vi "json_ltrim.vi"(10 "offset (0)":i32, 11 "data":string) -> (3 "left trim whitespace":string)   [LabVIEW 2017]
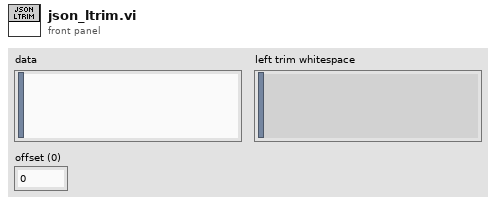
[diagram p1: front panel]
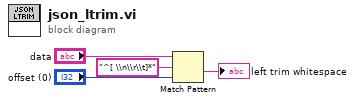
[diagram p0: block diagram]
diagram:
  n1 = Match Pattern(string="data", regular expression="^[ \\n\\r\\t]*", offset (0)="offset (0)") -> (after substring=→"left trim whitespace":string)  [unwired: 3 out]
